vi "pf_Scan_Ports.vi"(8 "error in (no error)":errorcluster) -> (0 "error out":errorcluster, 2 "Ports Info Array":T1[](array[typedef]))   [LabVIEW 2025, in "Photonfocus_Toolkit.lvlib"]
doc: "Executes a scan of the ports."
uses:
  Photonfocus_Toolkit.lvlib
  _Private/Controls/pf_Port_Info.ctl
  _Private/Controls/pf_CLALLSERIAL_Version.ctl
  _Private/Controls/pf_Port_Type.ctl
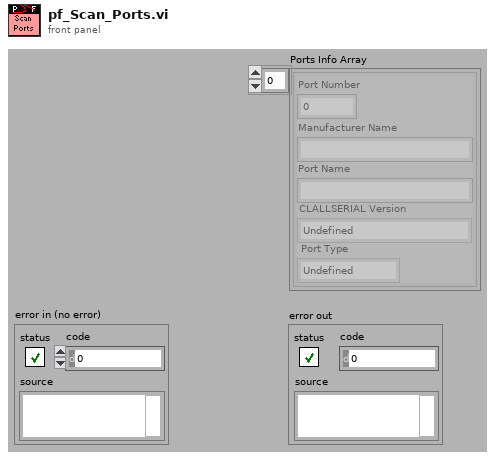
[diagram p1: front panel]
types:
  T1 = typedef "Photonfocus_Toolkit.lvlib/pf_Port_Info.ctl" = cluster{"Port Number":i32, "Manufacturer Name":string, "Port Name":string, "CLALLSERIAL Version":T2, "Port Type":T3}
  T2 = typedef "Photonfocus_Toolkit.lvlib/pf_CLALLSERIAL_Version.ctl" = enum16{"Undefined", "No CLALLSERIAL port", "CL_DLL_VERSION_NO_VERSION", "CL_DLL_VERSION_1_0", "CL_DLL_VERSION_1_1"}
  T3 = typedef "Photonfocus_Toolkit.lvlib/pf_Port_Type.ctl" = enum16{"Undefined", "CLALLSERIAL port", "port with clser.dll", "USB port", "RS-232 port"}
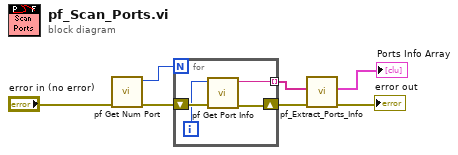
[diagram p0: block diagram]
diagram:
  n1 = call "pf Get Num Port.vi"("error in (no error)"="error in (no error)") -> ("error out"=w7:errorcluster, "function return"=w6:i32)  [unwired: 9 out]
  n2 = for {
    N: w6 -> [_]
    tunnel: [w10] -> w2 mode=indexing
    shift-right: [w9] -> w4
    shift-left: w7 -> [w11]
    i -> [w8]
    n3 = call "pf Get Port Info.vi"("error in (no error)"=w11, "iPort"=w8) -> ("error out"=w9:errorcluster, "function return"=w10:string)  [unwired: 8 out]
  }
  n4 = call "pf_Extract_Ports_Info.vi"("error in (no error)"=w4, "Ports Array"=w2) -> ("error out"=→"error out":errorcluster, "Ports Info Array"=→"Ports Info Array":T1[])  [unwired: 2 in, 6 out]
